vi "MIU_Control_v1.0.vi"() -> ()   [LabVIEW 2010]
uses:
  <vilib>/Utility/error.llb/DialogType.ctl
  <vilib>/Instr/_visa.llb/VISA Configure Serial Port (Instr).vi
  <vilib>/Analysis/NI_AALPro.lvlib
panel:
  in  "Tab Control":T1(tab)
  in  "Serial Read Port":refnum<visa-resource-name>="COM4"
  in  "data bits":u16=8 min=5 max=8 step=1
  in  "parity":u16(ring) items=["None", "Odd", "Even", "Mark", "Space"]
  in  "stop bits":u16(ring)=10 items=["1.0"=10, "1.5"=15, "2.0"=20]
  in  "flow control":u16(ring) items=["None"=0, "XON/XOFF"=1, "RTS/CTS"=2, "DTR/DSR"=4]
  in  "delay before read (ms)":u32=500
  in  "byte count":u32=500
  out "Incoming Serial String":string
  out "Time":string
  out "Date":string
  in  "Stop":bool
  out "return count":u32
  in  "Instrument baud rate (9600)":u32=9600
  in  "Control Port":refnum<visa-resource-name>="COM10"
  in  "Control baud rate":u32=9600
  out "N2O is FLAT":bool
  out "Rolling CO Slope Fit":cluster{i32[], "Best Linear Fit":dbl[]}[](graph)
  out "CO":dbl(graph)=0.310407
  out "N2O":dbl(graph)
  out "H2O":dbl(graph)
  out "CO PPM":string
  out "N2O PPM":string
  out "H2O PPM":string
  in  "Points to Average":i32
  out "CO Slope":dbl
  out "Rolling N2O Slope Fit 2":cluster{i32[], "Best Linear Fit":dbl[]}[](graph)
  out "N2O Slope":dbl
  in  "N2O Low Limit":dbl
  in  "CO High Limit":dbl
  out "CO is FLAT":bool
  in  "CO Low Limit":dbl
  in  "N2O High Limit":dbl
  out "Switch Valve":bool
  in  "Valve to switch":dbl min=0.0 max=16.0 step=1.0
  in  "Number of Bottles in Linearization":dbl=7.0
  out "?":bool
  out "Current Valve":dbl
  in  "Manually Switch Valves":bool
  out "Boolean":bool
  out "CELL TEMP":string
  out "CELL TEMPERATURE":dbl(graph)
  out "AMBIENT TEMPERATURE":dbl(graph)
  out "AMBIENT TEMP":string
  out "AIN5":dbl(graph)
  out "SUPERCOOL TEMP":string
  out "LINE LOCK":dbl(graph)
  out "LINELOCK - LASER CONTROL VOLTAGE":string
  out "PRESSURE":dbl(graph)
  out "PRESSURE 2":string
  out "SuperCool Temperature":dbl
  out "CO DRY 2":dbl(graph)
  out "N2O DRY":dbl(graph)
  out "CO DRY":string
  out "N2O DRY 2":string
  # "Automatic Linearization"
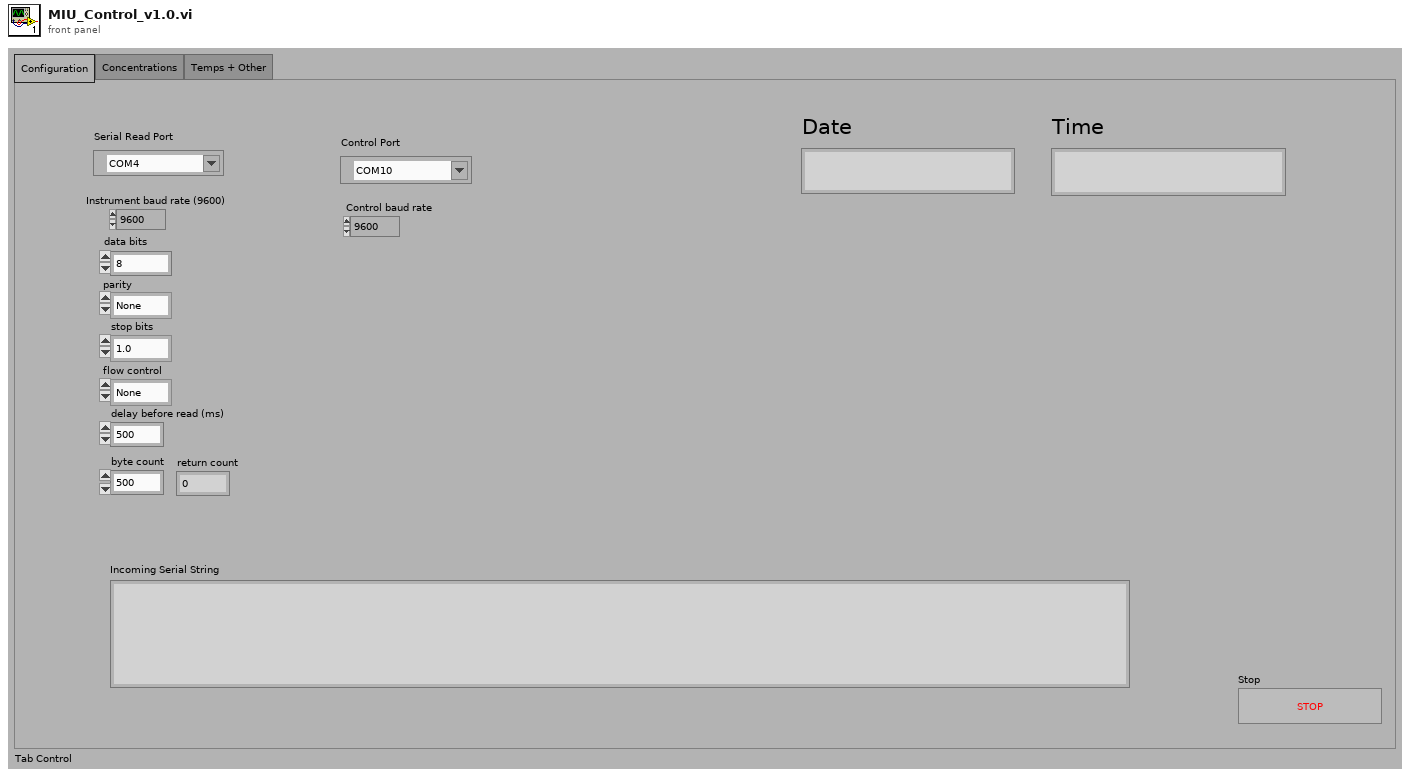
[diagram p1: front panel]
types:
  T1 = enum32{"Configuration", "Concentrations", "Temps + Other"}
  T2 = typedef "DialogType.ctl" = u16
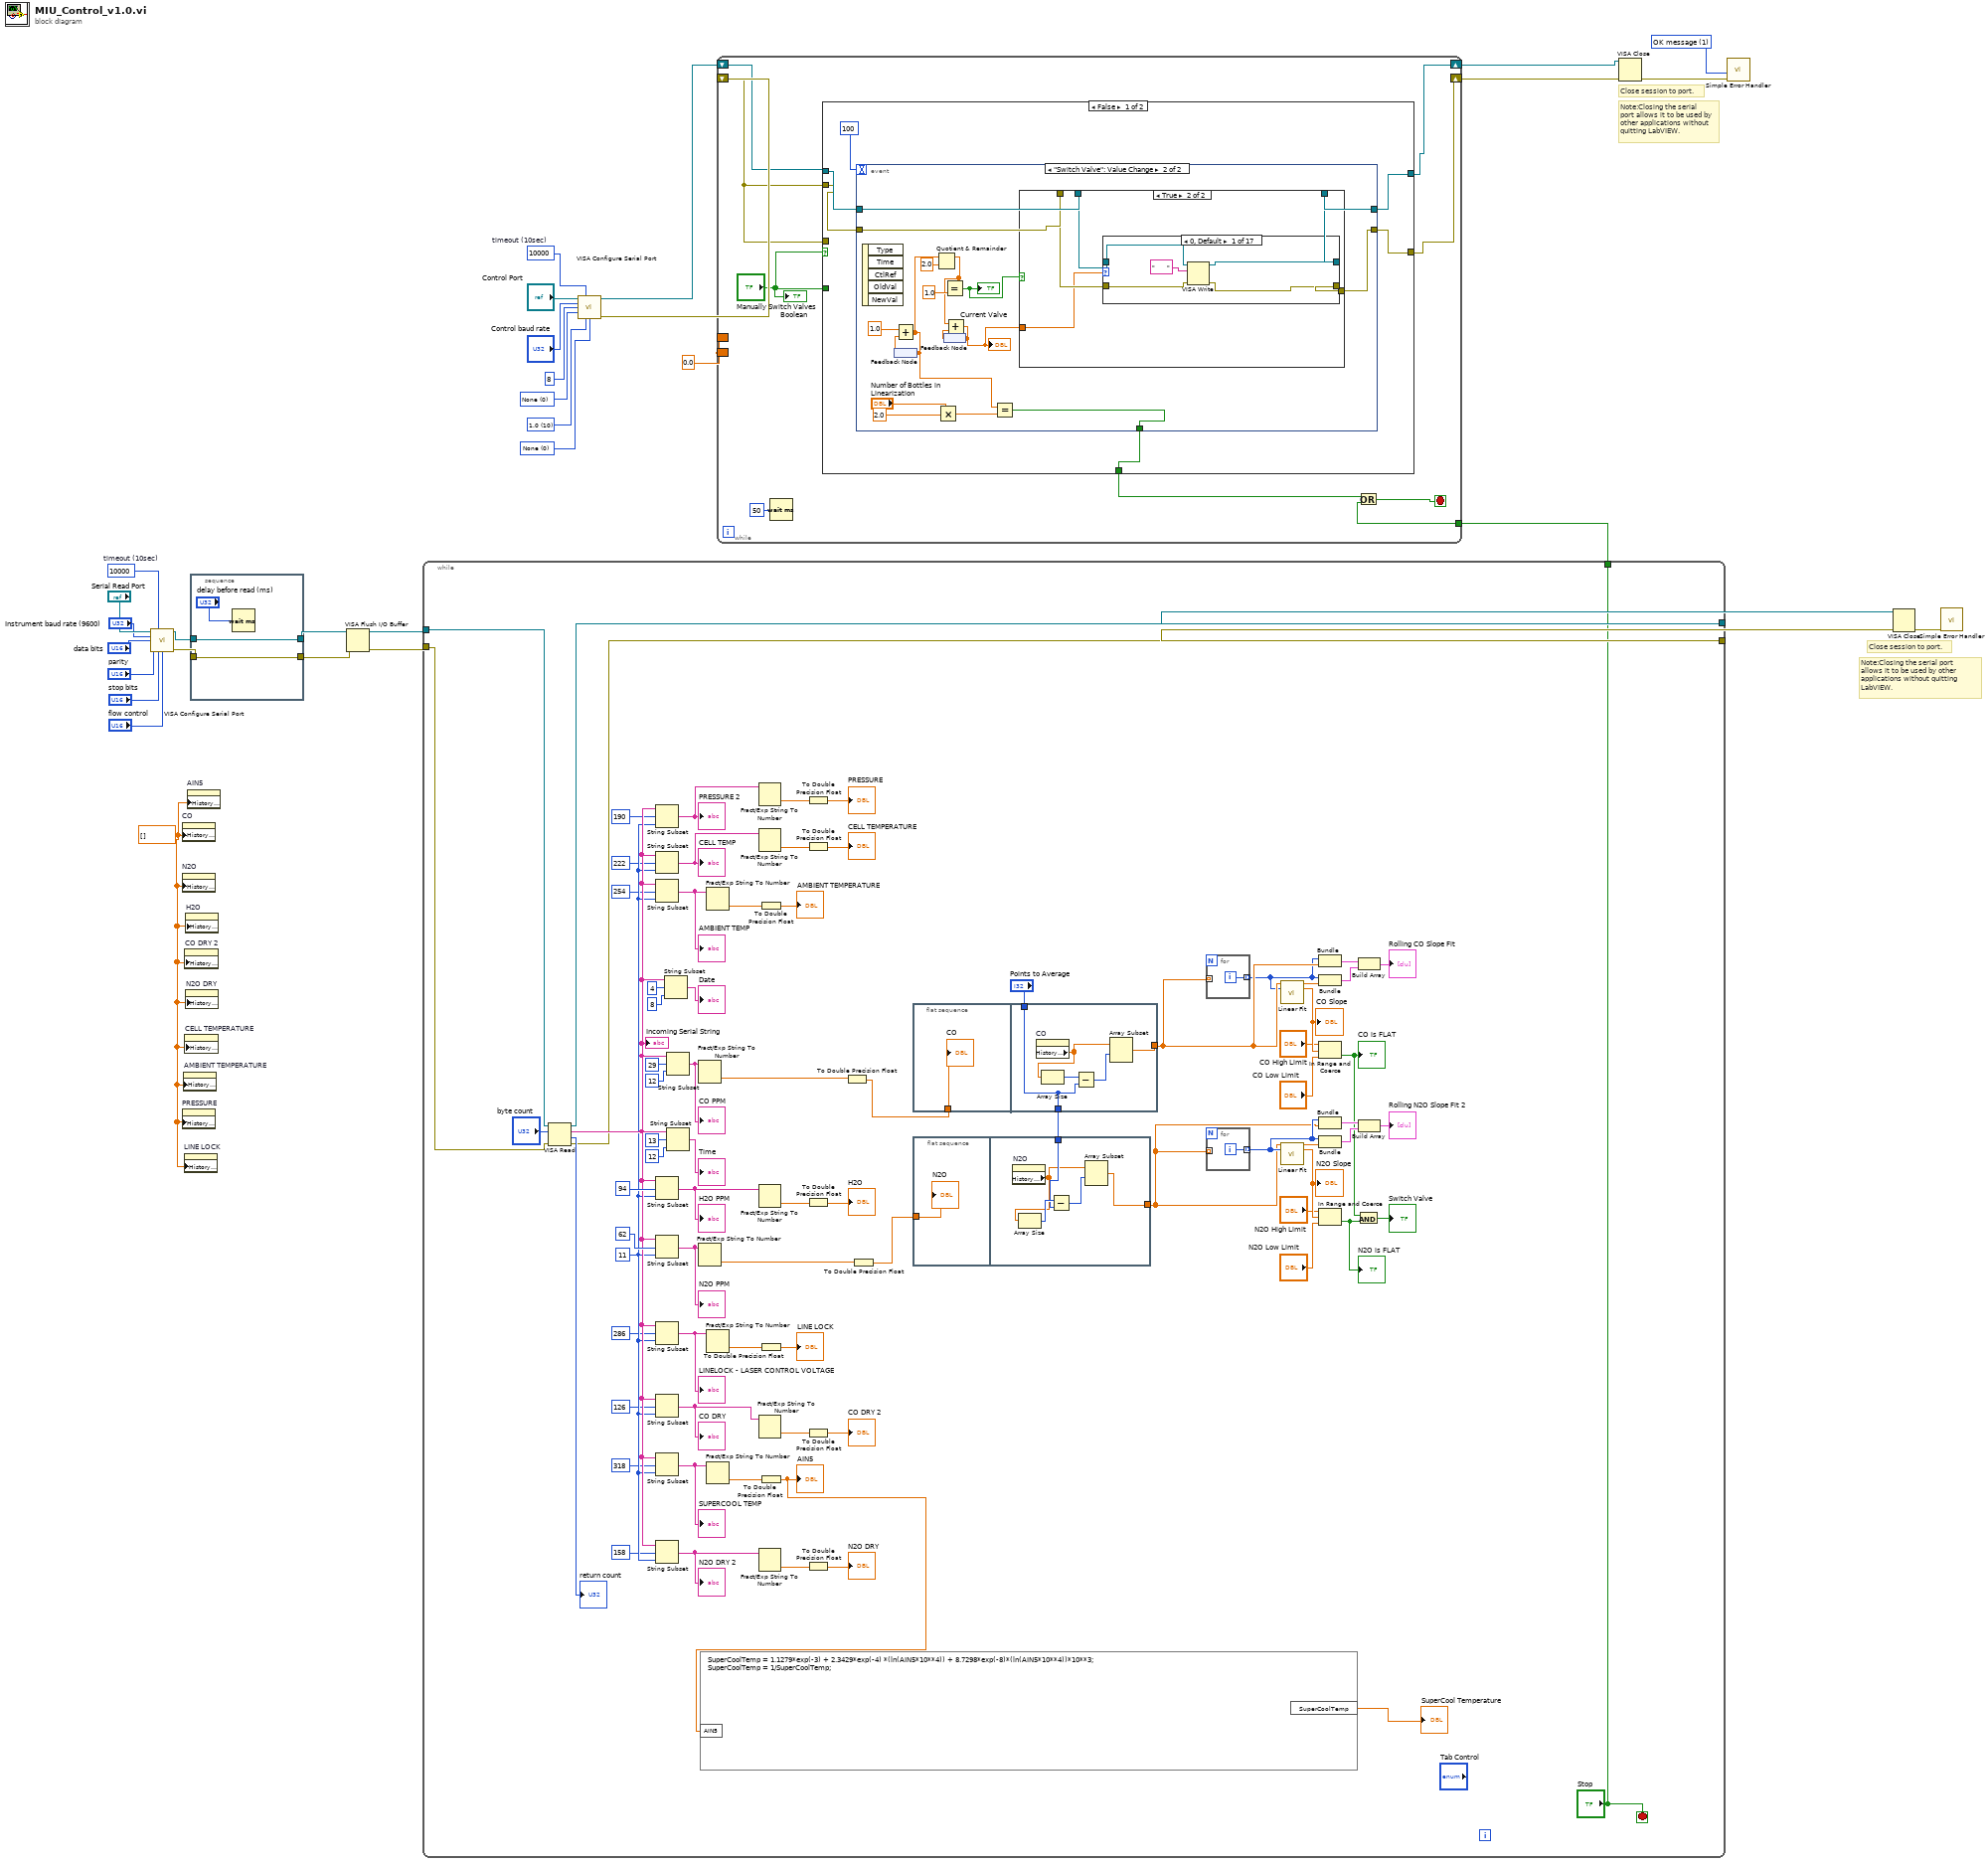
[diagram p0: block diagram]
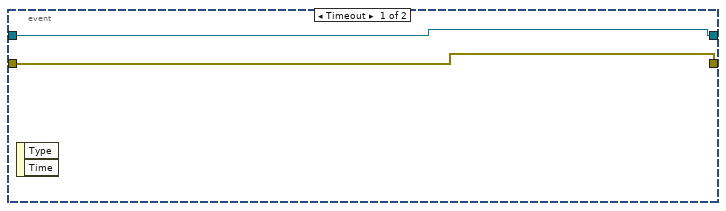
[diagram p2: hidden frame]
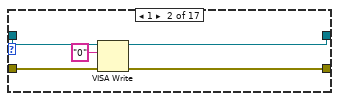
[diagram p4: hidden frame]
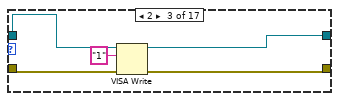
[diagram p5: hidden frame]
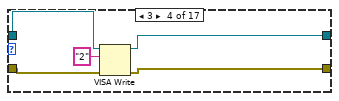
[diagram p6: hidden frame]
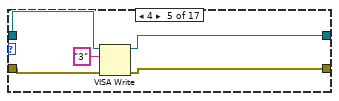
[diagram p7: hidden frame]
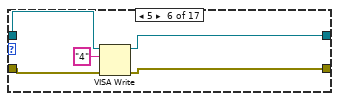
[diagram p8: hidden frame]
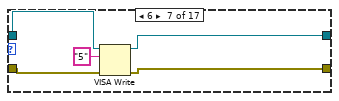
[diagram p9: hidden frame]
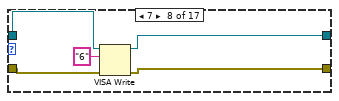
[diagram p10: hidden frame]
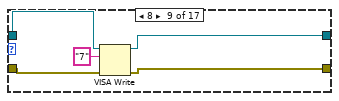
[diagram p11: hidden frame]
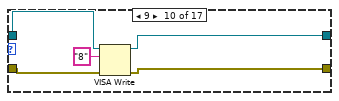
[diagram p12: hidden frame]
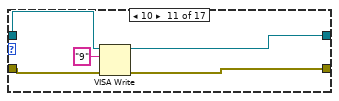
[diagram p13: hidden frame]
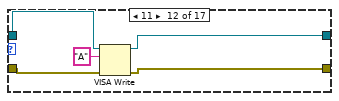
[diagram p14: hidden frame]
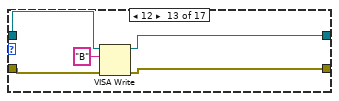
[diagram p15: hidden frame]
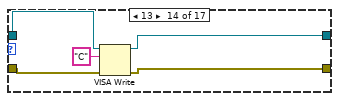
[diagram p16: hidden frame]
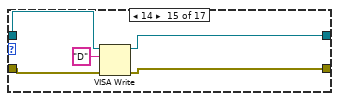
[diagram p17: hidden frame]
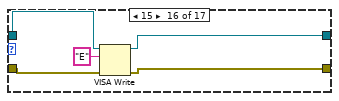
[diagram p18: hidden frame]
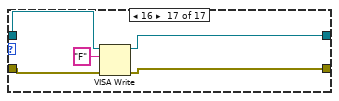
[diagram p19: hidden frame]
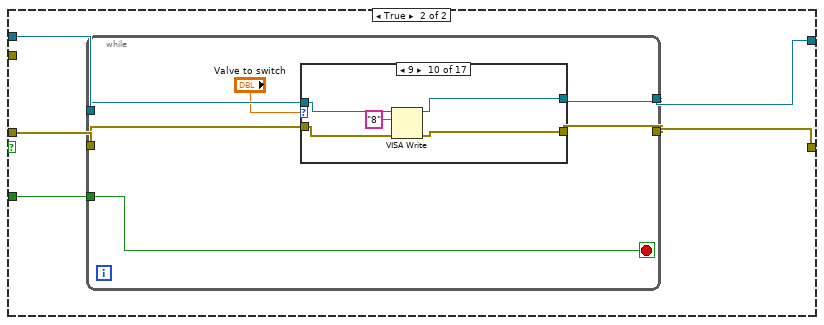
[diagram p20: hidden frame]
diagram:
  w2 = 0.0 ("Value (Signaling)")
  w6 = T2 1 items=["no dialog", "OK message", "continue or stop message", "OK message + warnings", "continue/stop + warnings"] ("type of dialog (OK msg:1)")
  w11 = u16 0 items=["None"=0, "XON/XOFF"=1, "RTS/CTS"=2, "DTR/DSR"=4] ("flow control")
  w12 = u16 10 items=["1.0"=10, "1.5"=15, "2.0"=20] ("stop bits")
  w14 = u16 0 items=["None", "Odd", "Even", "Mark", "Space"] ("parity")
  w13 = u32 10000  # timeout (10sec)
  w17 = dbl[] [] ("History Data")
  w29 = u32 10000  # timeout (10sec)
  # "Note:Closing the serial port allows it to be used by other applications without\nquitting LabVIEW."
  # "Close session to port."
  # "Note:Closing the serial port allows it to be used by other applications without quitting LabVIEW."
  # "Close session to port."
  n1 = call-poly "VISA Configure Serial Port"("VISA resource name"="Serial Read Port", "timeout (10sec)"=w29, "baud rate (9600)"="Instrument baud rate (9600)", "data bits (8)"="data bits", "parity (0:none)"="parity", "stop bits (10: 1 bit)"="stop bits", "flow control (0:none)"="flow control") -> ("VISA resource name out"=w24:refnum<visa-resource-name>, "error out"=w25:errorcluster)  [unwired: 2 in, 5 out]
  n2 = property on="CO" class="WFChart (strict)"("History Data"=w17) -> ()  [unwired: 2 in, 2 out]
  n3 = property on="N2O" class="WFChart (strict)"("History Data"=w17) -> ()  [unwired: 2 in, 2 out]
  n4 = property on="PRESSURE" class="WFChart (strict)"("History Data"=w17) -> ()  [unwired: 2 in, 2 out]
  n5 = property on="AMBIENT TEMPERATURE" class="WFChart (strict)"("History Data"=w17) -> ()  [unwired: 2 in, 2 out]
  n6 = property on="LINE LOCK" class="WFChart (strict)"("History Data"=w17) -> ()  [unwired: 2 in, 2 out]
  n7 = property on="CO DRY 2" class="WFChart (strict)"("History Data"=w17) -> ()  [unwired: 2 in, 2 out]
  n8 = property on="CELL TEMPERATURE" class="WFChart (strict)"("History Data"=w17) -> ()  [unwired: 2 in, 2 out]
  n9 = property on="H2O" class="WFChart (strict)"("History Data"=w17) -> ()  [unwired: 2 in, 2 out]
  n10 = property on="N2O DRY" class="WFChart (strict)"("History Data"=w17) -> ()  [unwired: 2 in, 2 out]
  n11 = property on="AIN5" class="WFChart (strict)"("History Data"=w17) -> ()  [unwired: 2 in, 2 out]
  n12 = stacked-sequence {
    tunnel: w25 -> [w35]
    tunnel: [w35] -> w18
    tunnel: w24 -> [w34]
    tunnel: [w34] -> w19
    frame #0 {
      n13 = Wait (ms)(milliseconds to wait="delay before read (ms)") -> ()  [unwired: 1 out]
    }
  }
  n14 = VISA Flush I/O Buffer(VISA resource name=w19, error in (no error)=w18) -> (VISA resource name out=w21:refnum<visa-resource-name>, error out=w20:errorcluster)  [unwired: 1 in]
  n15 = while {
    tunnel: w21 -> [w85]
    tunnel: w20 -> [w86]
    tunnel: [w108] -> w23
    tunnel: [w64] -> w22
    tunnel: ["Stop"] -> w1
    stop <- "Stop" stop-if-true
    w75 = 11 ("offset (0)")
    n16 = VISA Read(VISA resource name=w85, byte count="byte count", error in (no error)=w86) -> (VISA resource name out=w108:refnum<visa-resource-name>, read buffer=w76:string, return count=→"return count":u32, error out=w64:errorcluster)
    "Incoming Serial String" <- w76
    n17 = String Subset(string=w76, offset (0)=190, length (rest)=w75) -> (substring=w88:string)
    "PRESSURE 2" <- w88
    n18 = String Subset(string=w76, offset (0)=222, length (rest)=w75) -> (substring=w87:string)
    "CELL TEMP" <- w87
    n19 = String Subset(string=w76, offset (0)=254, length (rest)=w75) -> (substring=w79:string)
    "AMBIENT TEMP" <- w79
    n20 = String Subset(string=w76, offset (0)=94, length (rest)=w75) -> (substring=w101:string)
    "H2O PPM" <- w101
    n21 = String Subset(string=w76, offset (0)=62, length (rest)=w75) -> (substring=w102:string)
    "N2O PPM" <- w102
    n22 = String Subset(string=w76, offset (0)=286, length (rest)=w75) -> (substring=w78:string)
    "LINELOCK - LASER CONTROL VOLTAGE" <- w78
    n23 = String Subset(string=w76, offset (0)=126, length (rest)=w75) -> (substring=w90:string)
    "CO DRY" <- w90
    n24 = String Subset(string=w76, offset (0)=318, length (rest)=w75) -> (substring=w77:string)
    "SUPERCOOL TEMP" <- w77
    n25 = String Subset(string=w76, offset (0)=158, length (rest)=w75) -> (substring=w89:string)
    "N2O DRY 2" <- w89
    n26 = String Subset(string=w76, offset (0)=4, length (rest)=8 ("length (rest)")) -> (substring=→"Date":string)
    n27 = String Subset(string=w76, offset (0)=29, length (rest)=12 ("length (rest)")) -> (substring=w103:string)
    "CO PPM" <- w103
    n28 = String Subset(string=w76, offset (0)=13, length (rest)=12 ("length (rest)")) -> (substring=→"Time":string)
    n29 = Fract/Exp String To Number(string=w103) -> (number=w100:dbl)  [unwired: 3 in, 1 out]
    n30 = Fract/Exp String To Number(string=w102) -> (number=w56:dbl)  [unwired: 3 in, 1 out]
    n31 = Fract/Exp String To Number(string=w79) -> (number=w83:dbl)  [unwired: 3 in, 1 out]
    n32 = Fract/Exp String To Number(string=w78) -> (number=w81:dbl)  [unwired: 3 in, 1 out]
    n33 = Fract/Exp String To Number(string=w77) -> (number=w80:dbl)  [unwired: 3 in, 1 out]
    n34 = Fract/Exp String To Number(string=w88) -> (number=w93:dbl)  [unwired: 3 in, 1 out]
    n35 = Fract/Exp String To Number(string=w87) -> (number=w91:dbl)  [unwired: 3 in, 1 out]
    n36 = Fract/Exp String To Number(string=w101) -> (number=w99:dbl)  [unwired: 3 in, 1 out]
    n37 = Fract/Exp String To Number(string=w90) -> (number=w97:dbl)  [unwired: 3 in, 1 out]
    n38 = Fract/Exp String To Number(string=w89) -> (number=w95:dbl)  [unwired: 3 in, 1 out]
    n39 = To Double Precision Float(number=w83) -> (double precision float=→"AMBIENT TEMPERATURE":dbl)
    n40 = To Double Precision Float(number=w81) -> (double precision float=→"LINE LOCK":dbl)
    n41 = To Double Precision Float(number=w80) -> (double precision float=w36:dbl)
    "AIN5" <- w36
    n42 = formula code="SuperCoolTemp = 1.1279*exp(-3) + 2.3429*exp(-4) *(ln(AIN5*10**4)) + 8.7298*exp(-8)*(ln(AIN5*10**4))*10**3;\nSuperCoolTemp = 1/SuperCoolTemp;"("AIN5"=w36) -> ("SuperCoolTemp"=→"SuperCool Temperature":dbl)
    n43 = To Double Precision Float(number=w93) -> (double precision float=→"PRESSURE":dbl)
    n44 = To Double Precision Float(number=w91) -> (double precision float=→"CELL TEMPERATURE":dbl)
    n45 = To Double Precision Float(number=w99) -> (double precision float=→"H2O":dbl)
    n46 = To Double Precision Float(number=w97) -> (double precision float=→"CO DRY 2":dbl)
    n47 = To Double Precision Float(number=w95) -> (double precision float=→"N2O DRY":dbl)
    n48 = To Double Precision Float(number=w100) -> (double precision float=w63:dbl)
    n49 = To Double Precision Float(number=w56) -> (double precision float=w55:dbl)
    n50 = flat-sequence {
      tunnel: w63 -> [w124]
      tunnel: [w126] -> w62
      tunnel: "Points to Average" -> [w125]
      tunnel: [w125] -> w53
      frame #0 {
        "CO" <- w124
      }
      frame #1 {
        n51 = property on="CO" class="WFChart (strict)"() -> ("History Data"=w127:dbl[])  [unwired: 2 in, 2 out]
        n52 = Array Size(array=w127) -> (size(s)=w128:i32)
        n53 = Subtract(x=w128, y=w125) -> (x-y=w129:i32)
        n54 = Array Subset(array=w127, index=w129) -> (w126:dbl[])  [unwired: 1 in]
      }
    }
    n55 = flat-sequence {
      tunnel: w55 -> [w117]
      tunnel: w53 -> [w120]
      tunnel: [w118] -> w47
      frame #0 {
        "N2O" <- w117
      }
      frame #1 {
        n56 = property on="N2O" class="WFChart (strict)"() -> ("History Data"=w119:dbl[])  [unwired: 2 in, 2 out]
        n57 = Array Size(array=w119) -> (size(s)=w121:i32)
        n58 = Subtract(x=w121, y=w120) -> (x-y=w122:i32)
        n59 = Array Subset(array=w119, index=w122) -> (w118:dbl[])  [unwired: 1 in]
      }
    }
    n60 = for {
      tunnel: [w123] -> w61 mode=indexing
      tunnel: w62 -> [_] mode=indexing
      i -> [w123]
    }
    n61 = for {
      tunnel: [w116] -> w52 mode=indexing
      tunnel: w47 -> [_] mode=indexing
      i -> [w116]
    }
    n62 = call <vilib>:"Linear Fit.vi"("Y"=w62, "X"=w61) -> ("Best Linear Fit"=w60:dbl[], "slope"=w46:dbl)  [unwired: 9 in, 3 out]
    "CO Slope" <- w46
    n63 = call <vilib>:"Linear Fit.vi"("Y"=w47, "X"=w52) -> ("Best Linear Fit"=w51:dbl[], "slope"=w43:dbl)  [unwired: 9 in, 3 out]
    "N2O Slope" <- w43
    n64 = Bundle(w61, w62) -> (w59:cluster{i32[], dbl[]})  [unwired: 1 in]
    n65 = Bundle(w61, "Best Linear Fit"=w60) -> (w58:cluster{i32[], "Best Linear Fit":dbl[]})  [unwired: 1 in]
    n66 = In Range and Coerce(upper limit="CO High Limit", x=w46, lower limit="CO Low Limit") -> (In Range?=w40:bool)  [unwired: 1 out]
    "CO is FLAT" <- w40
    n67 = Bundle(w52, w47) -> (w50:cluster{i32[], dbl[]})  [unwired: 1 in]
    n68 = Bundle(w52, "Best Linear Fit"=w51) -> (w49:cluster{i32[], "Best Linear Fit":dbl[]})  [unwired: 1 in]
    n69 = In Range and Coerce(upper limit="N2O High Limit", x=w43, lower limit="N2O Low Limit") -> (In Range?=w39:bool)  [unwired: 1 out]
    "N2O is FLAT" <- w39
    n70 = And(x=w40, y=w39) -> (x .and. y?=→"Switch Valve":bool)
    n71 = Build Array(w59, w58) -> (→"Rolling CO Slope Fit":cluster{i32[], "Best Linear Fit":dbl[]}[])
    n72 = Build Array(w50, w49) -> (→"Rolling N2O Slope Fit 2":cluster{i32[], "Best Linear Fit":dbl[]}[])
  }
  n73 = call-poly "VISA Configure Serial Port"("VISA resource name"="Control Port", "timeout (10sec)"=w13, "baud rate (9600)"="Control baud rate", "data bits (8)"=u16 8 ("data bits"), "parity (0:none)"=w14, "stop bits (10: 1 bit)"=w12, "flow control (0:none)"=w11) -> ("VISA resource name out"=w5:refnum<visa-resource-name>, "error out"=w3:errorcluster)  [unwired: 2 in, 5 out]
  n74 = while {
    shift-right: [w136] -> w4
    shift-left: w3 -> [w135]
    shift-right: [w137] -> w7
    shift-left: w5 -> [w138]
    border: w2 -> [_]
    border: w2 -> [_]
    tunnel: w1 -> [w130]
    stop <- w132 stop-if-true
    n75 = Wait (ms)(milliseconds to wait=u32 50) -> ()  [unwired: 1 out]
    n76 = case shown="False" "Manually Switch Valves" {
      tunnel: w138 -> [w142 w260]
      tunnel: w135 -> [_ w259]
      tunnel: [w141 w257] -> w137
      tunnel: [w140 w256] -> w136
      tunnel: w135 -> [w139 _]
      tunnel: "Manually Switch Valves" -> [_ w258]
      tunnel: [w144 _] -> w133
      frame False {
        n77 = event shown="[1] \"Switch Valve\": Value Change" {
          selector: _ -> [_ _]
          dyn-events: _ -> [_ _]
          timeout: 100 -> [_ _]
          tunnel: [_ w147] -> w144
          tunnel: [w146 w156] -> w141
          tunnel: w142 -> [w146 w158]
          tunnel: w139 -> [w145 w157]
          tunnel: [w145 w155] -> w140
          event Timeout {
            n78 = event-data() -> ()  [unwired: 1 in, 2 out]
          }
          event "Switch Valve": Value Change {
            n79 = event-data() -> ()  [unwired: 1 in, 5 out]
            n80 = feedback #1() -> (w163:dbl)
            n81 = Add(x=1.0, y=w163) -> (x+y=w154:dbl)
            n82 = feedback-in #1(w154) -> ()
            n83 = Quotient & Remainder(x=w154, y=2.0) -> (x-y*floor(x/y)=w152:dbl)  [unwired: 1 out]
            n84 = Multiply(x="Number of Bottles in Linearization", y=2.0) -> (x*y=w148:dbl)
            n85 = Equal?(x=w152, y=1.0) -> (x = y?=w159:bool)
            "?" <- w159
            n86 = feedback #2() -> (w153:dbl)
            n87 = Add(x=w152, y=w153) -> (x+y=w151:dbl)
            "Current Valve" <- w151
            n88 = feedback-in #2(w151) -> ()
            n89 = Equal?(x=w154, y=w148) -> (x = y?=w147:bool)
            n90 = case shown="True" w159 {
              tunnel: w158 -> [w164 w170]
              tunnel: w157 -> [w165 w169]
              tunnel: [w164 w168] -> w156
              tunnel: [w165 w167] -> w155
              tunnel: w151 -> [_ w166]
              frame False {
              }
              frame True {
                n91 = case shown="0, Default" w166 {
                  tunnel: [w174 w180 w184 w189 w194 w199 w204 w209 w214 w219 w222 w229 w234 w239 w244 w249 w254] -> w168
                  tunnel: [w173 w179 w183 w188 w193 w198 w203 w208 w213 w218 w221 w228 w233 w238 w243 w248 w253] -> w167
                  tunnel: w170 -> [w172 w177 w182 w187 w192 w197 w202 w207 w212 w217 w224 w227 w232 w237 w242 w247 w252]
                  tunnel: w169 -> [w171 w176 w181 w186 w191 w196 w201 w206 w211 w216 w223 w226 w231 w236 w241 w246 w251]
                  frame 0, Default {
                    n92 = VISA Write(VISA resource name=w172, write buffer="      ", error in (no error)=w171) -> (VISA resource name out=w174:refnum<visa-resource-name>, error out=w173:errorcluster)  [unwired: 1 out]
                  }
                  frame 1 {
                    n93 = VISA Write(VISA resource name=w177, write buffer="0", error in (no error)=w176) -> (VISA resource name out=w180:refnum<visa-resource-name>, error out=w179:errorcluster)  [unwired: 1 out]
                  }
                  frame 2 {
                    n94 = VISA Write(VISA resource name=w182, write buffer="1", error in (no error)=w181) -> (VISA resource name out=w184:refnum<visa-resource-name>, error out=w183:errorcluster)  [unwired: 1 out]
                  }
                  frame 3 {
                    n95 = VISA Write(VISA resource name=w187, write buffer="2", error in (no error)=w186) -> (VISA resource name out=w189:refnum<visa-resource-name>, error out=w188:errorcluster)  [unwired: 1 out]
                  }
                  frame 4 {
                    n96 = VISA Write(VISA resource name=w192, write buffer="3", error in (no error)=w191) -> (VISA resource name out=w194:refnum<visa-resource-name>, error out=w193:errorcluster)  [unwired: 1 out]
                  }
                  frame 5 {
                    n97 = VISA Write(VISA resource name=w197, write buffer="4", error in (no error)=w196) -> (VISA resource name out=w199:refnum<visa-resource-name>, error out=w198:errorcluster)  [unwired: 1 out]
                  }
                  frame 6 {
                    n98 = VISA Write(VISA resource name=w202, write buffer="5", error in (no error)=w201) -> (VISA resource name out=w204:refnum<visa-resource-name>, error out=w203:errorcluster)  [unwired: 1 out]
                  }
                  frame 7 {
                    n99 = VISA Write(VISA resource name=w207, write buffer="6", error in (no error)=w206) -> (VISA resource name out=w209:refnum<visa-resource-name>, error out=w208:errorcluster)  [unwired: 1 out]
                  }
                  frame 8 {
                    n100 = VISA Write(VISA resource name=w212, write buffer="7", error in (no error)=w211) -> (VISA resource name out=w214:refnum<visa-resource-name>, error out=w213:errorcluster)  [unwired: 1 out]
                  }
                  frame 9 {
                    n101 = VISA Write(VISA resource name=w217, write buffer="8", error in (no error)=w216) -> (VISA resource name out=w219:refnum<visa-resource-name>, error out=w218:errorcluster)  [unwired: 1 out]
                  }
                  frame 10 {
                    n102 = VISA Write(VISA resource name=w224, write buffer="9", error in (no error)=w223) -> (VISA resource name out=w222:refnum<visa-resource-name>, error out=w221:errorcluster)  [unwired: 1 out]
                  }
                  frame 11 {
                    n103 = VISA Write(VISA resource name=w227, write buffer="A", error in (no error)=w226) -> (VISA resource name out=w229:refnum<visa-resource-name>, error out=w228:errorcluster)  [unwired: 1 out]
                  }
                  frame 12 {
                    n104 = VISA Write(VISA resource name=w232, write buffer="B", error in (no error)=w231) -> (VISA resource name out=w234:refnum<visa-resource-name>, error out=w233:errorcluster)  [unwired: 1 out]
                  }
                  frame 13 {
                    n105 = VISA Write(VISA resource name=w237, write buffer="C", error in (no error)=w236) -> (VISA resource name out=w239:refnum<visa-resource-name>, error out=w238:errorcluster)  [unwired: 1 out]
                  }
                  frame 14 {
                    n106 = VISA Write(VISA resource name=w242, write buffer="D", error in (no error)=w241) -> (VISA resource name out=w244:refnum<visa-resource-name>, error out=w243:errorcluster)  [unwired: 1 out]
                  }
                  frame 15 {
                    n107 = VISA Write(VISA resource name=w247, write buffer="E", error in (no error)=w246) -> (VISA resource name out=w249:refnum<visa-resource-name>, error out=w248:errorcluster)  [unwired: 1 out]
                  }
                  frame 16 {
                    n108 = VISA Write(VISA resource name=w252, write buffer="F", error in (no error)=w251) -> (VISA resource name out=w254:refnum<visa-resource-name>, error out=w253:errorcluster)  [unwired: 1 out]
                  }
                }
              }
            }
          }
        }
      }
      frame True {
        n109 = while {
          tunnel: w260 -> [w265]
          tunnel: w259 -> [w264]
          tunnel: w258 -> [w266]
          tunnel: [w262] -> w257
          tunnel: [w261] -> w256
          stop <- w266 stop-if-true
          n110 = case shown="9" "Valve to switch" {
            tunnel: [w270 w276 w280 w285 w290 w295 w300 w305 w310 w315 w320 w325 w330 w335 w340 w345 w350] -> w262
            tunnel: [w269 w275 w279 w284 w289 w294 w299 w304 w309 w314 w319 w324 w329 w334 w339 w344 w349] -> w261
            tunnel: w265 -> [w268 w273 w278 w283 w288 w293 w298 w303 w308 w313 w318 w323 w328 w333 w338 w343 w348]
            tunnel: w264 -> [w267 w272 w277 w282 w287 w292 w297 w302 w307 w312 w317 w322 w327 w332 w337 w342 w347]
            frame 0, Default {
              n111 = VISA Write(VISA resource name=w268, write buffer="      ", error in (no error)=w267) -> (VISA resource name out=w270:refnum<visa-resource-name>, error out=w269:errorcluster)  [unwired: 1 out]
            }
            frame 1 {
              n112 = VISA Write(VISA resource name=w273, write buffer="0", error in (no error)=w272) -> (VISA resource name out=w276:refnum<visa-resource-name>, error out=w275:errorcluster)  [unwired: 1 out]
            }
            frame 2 {
              n113 = VISA Write(VISA resource name=w278, write buffer="1", error in (no error)=w277) -> (VISA resource name out=w280:refnum<visa-resource-name>, error out=w279:errorcluster)  [unwired: 1 out]
            }
            frame 3 {
              n114 = VISA Write(VISA resource name=w283, write buffer="2", error in (no error)=w282) -> (VISA resource name out=w285:refnum<visa-resource-name>, error out=w284:errorcluster)  [unwired: 1 out]
            }
            frame 4 {
              n115 = VISA Write(VISA resource name=w288, write buffer="3", error in (no error)=w287) -> (VISA resource name out=w290:refnum<visa-resource-name>, error out=w289:errorcluster)  [unwired: 1 out]
            }
            frame 5 {
              n116 = VISA Write(VISA resource name=w293, write buffer="4", error in (no error)=w292) -> (VISA resource name out=w295:refnum<visa-resource-name>, error out=w294:errorcluster)  [unwired: 1 out]
            }
            frame 6 {
              n117 = VISA Write(VISA resource name=w298, write buffer="5", error in (no error)=w297) -> (VISA resource name out=w300:refnum<visa-resource-name>, error out=w299:errorcluster)  [unwired: 1 out]
            }
            frame 7 {
              n118 = VISA Write(VISA resource name=w303, write buffer="6", error in (no error)=w302) -> (VISA resource name out=w305:refnum<visa-resource-name>, error out=w304:errorcluster)  [unwired: 1 out]
            }
            frame 8 {
              n119 = VISA Write(VISA resource name=w308, write buffer="7", error in (no error)=w307) -> (VISA resource name out=w310:refnum<visa-resource-name>, error out=w309:errorcluster)  [unwired: 1 out]
            }
            frame 9 {
              n120 = VISA Write(VISA resource name=w313, write buffer="8", error in (no error)=w312) -> (VISA resource name out=w315:refnum<visa-resource-name>, error out=w314:errorcluster)  [unwired: 1 out]
            }
            frame 10 {
              n121 = VISA Write(VISA resource name=w318, write buffer="9", error in (no error)=w317) -> (VISA resource name out=w320:refnum<visa-resource-name>, error out=w319:errorcluster)  [unwired: 1 out]
            }
            frame 11 {
              n122 = VISA Write(VISA resource name=w323, write buffer="A", error in (no error)=w322) -> (VISA resource name out=w325:refnum<visa-resource-name>, error out=w324:errorcluster)  [unwired: 1 out]
            }
            frame 12 {
              n123 = VISA Write(VISA resource name=w328, write buffer="B", error in (no error)=w327) -> (VISA resource name out=w330:refnum<visa-resource-name>, error out=w329:errorcluster)  [unwired: 1 out]
            }
            frame 13 {
              n124 = VISA Write(VISA resource name=w333, write buffer="C", error in (no error)=w332) -> (VISA resource name out=w335:refnum<visa-resource-name>, error out=w334:errorcluster)  [unwired: 1 out]
            }
            frame 14 {
              n125 = VISA Write(VISA resource name=w338, write buffer="D", error in (no error)=w337) -> (VISA resource name out=w340:refnum<visa-resource-name>, error out=w339:errorcluster)  [unwired: 1 out]
            }
            frame 15 {
              n126 = VISA Write(VISA resource name=w343, write buffer="E", error in (no error)=w342) -> (VISA resource name out=w345:refnum<visa-resource-name>, error out=w344:errorcluster)  [unwired: 1 out]
            }
            frame 16 {
              n127 = VISA Write(VISA resource name=w348, write buffer="F", error in (no error)=w347) -> (VISA resource name out=w350:refnum<visa-resource-name>, error out=w349:errorcluster)  [unwired: 1 out]
            }
          }
        }
      }
    }
    n128 = Or(x=w133, y=w130) -> (x .or. y?=w132:bool)
    "Boolean" <- "Manually Switch Valves"
  }
  n129 = VISA Close(VISA resource name=w7, error in (no error)=w4) -> (error out=w9:errorcluster)
  n130 = call <vilib>:"Simple Error Handler.vi"("type of dialog (OK msg:1)"=w6, "error in (no error)"=w9) -> ()  [unwired: 8 out]
  n131 = VISA Close(VISA resource name=w23, error in (no error)=w22) -> (error out=w31:errorcluster)
  n132 = call <vilib>:"Simple Error Handler.vi"("error in (no error)"=w31) -> ()  [unwired: 1 in, 8 out]
